vi "About.vi"() -> ()   [LabVIEW 2015]
uses:
  <vilib>/Platform/browser.llb/Open URL in Default Browser (string).vi
  GlobalVar.vi
panel:
  in  "btnReg":bool
  out "txtCopyright":string="版权归许晓通所有,欢迎个人转发分享。"
  out "txtContact":string="如有其它疑问，欢迎私信留言或联系QQ：19627152   QQ群：646900507。"
  out "txtXCANdeveloper":string="作者：Jay Sur (许晓通) @华南理工大学"
  out "txtXCAN":string="X-CAN离线分析平台"
  out "JayWeb":string
  in  "GoJayWeb":bool
  out "txtshowSupportFormat":string caption="The file format supported:"
  in  "btnGoBlog":bool
  in  "btnClose":bool
  out "UserGroup":string caption="用户组:"
  out "CurVersion":string caption="Version:"
  out "HelpBlogURL":string caption="Introduction and help, please see:"
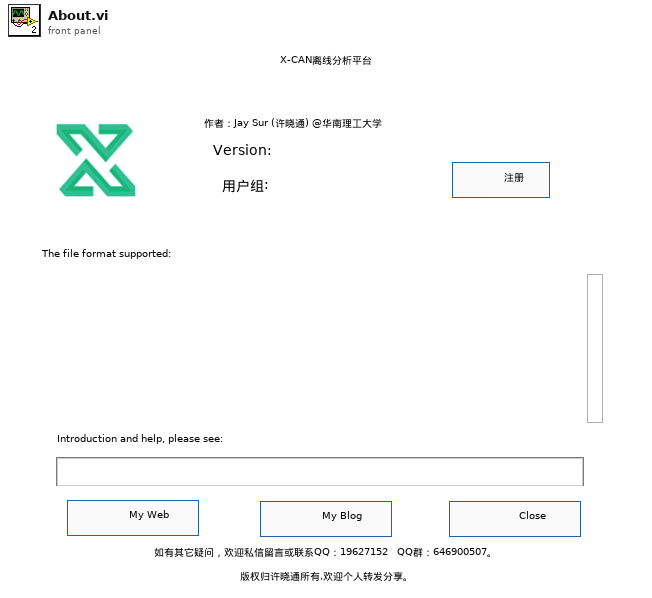
[diagram p1: front panel]
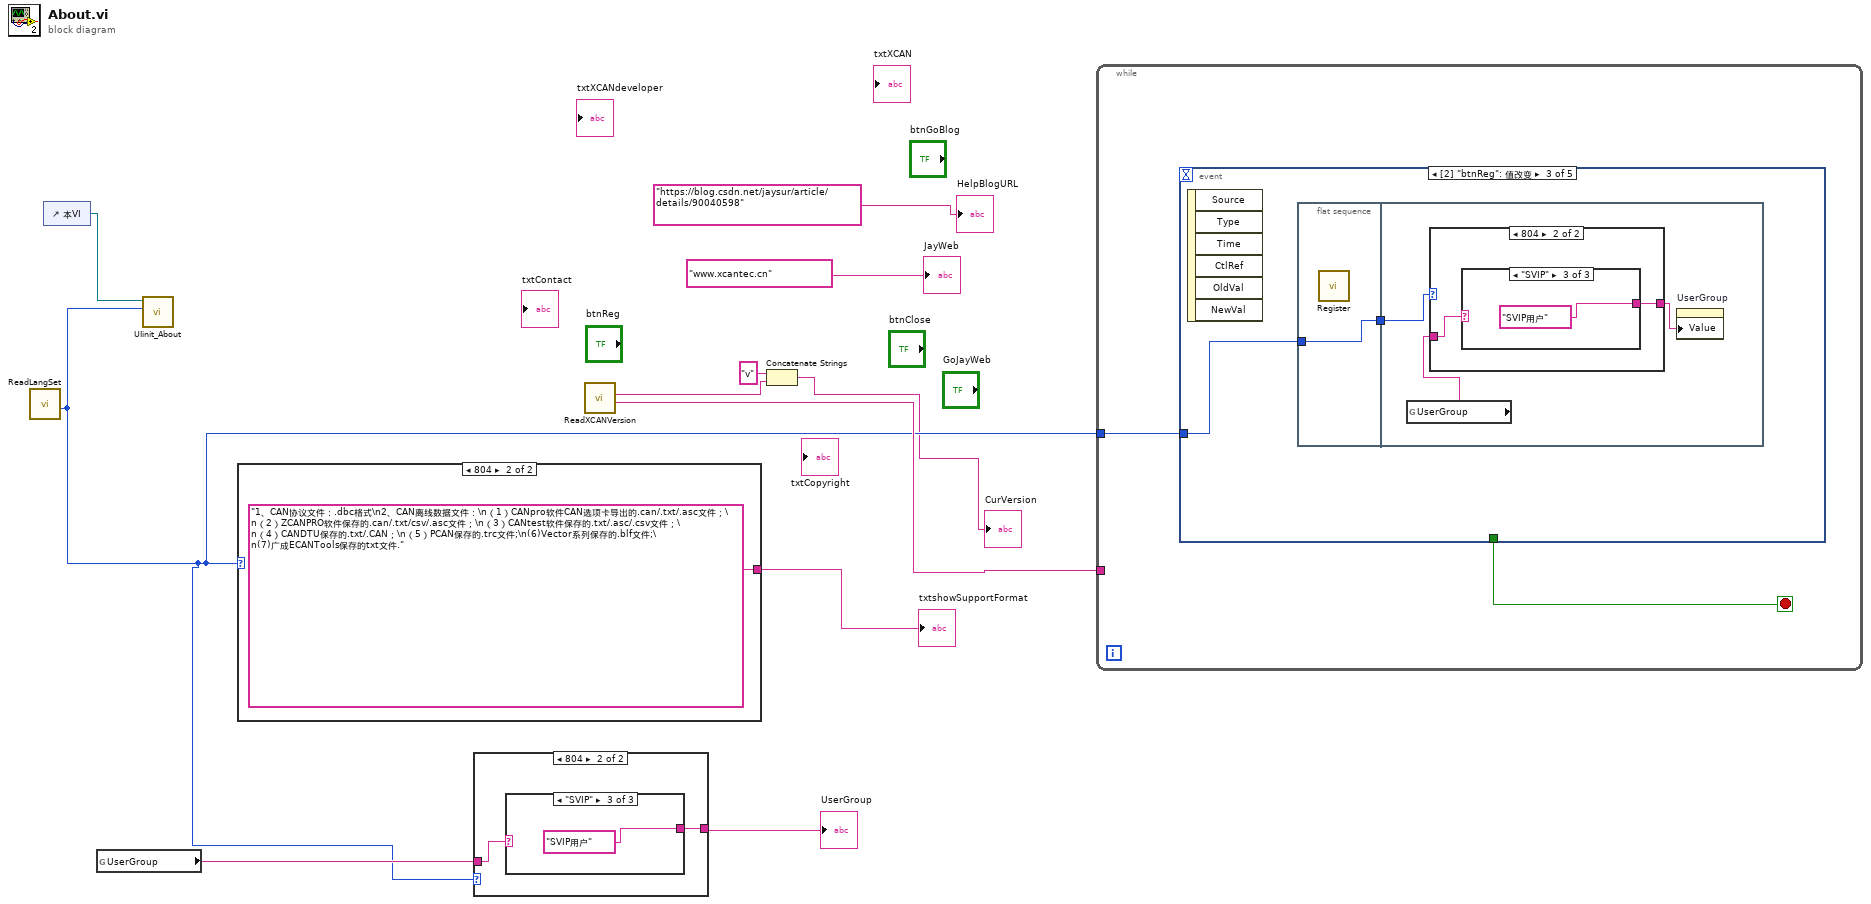
[diagram p0: block diagram]
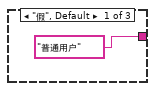
[diagram p3: hidden frame]
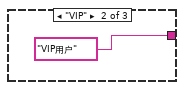
[diagram p4: hidden frame]
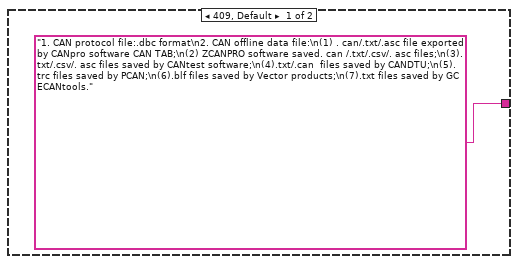
[diagram p5: hidden frame]
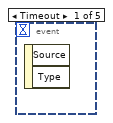
[diagram p6: hidden frame]
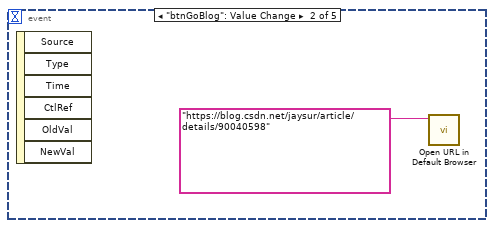
[diagram p7: hidden frame]
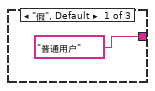
[diagram p9: hidden frame]
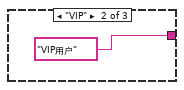
[diagram p10: hidden frame]
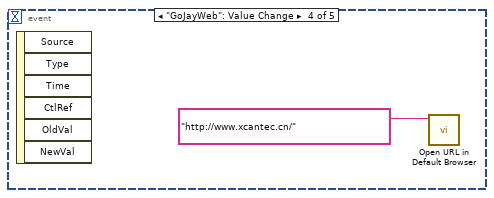
[diagram p11: hidden frame]
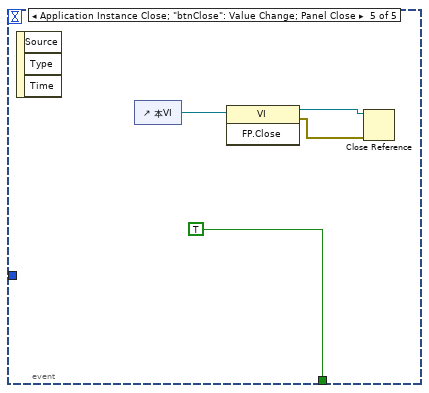
[diagram p12: hidden frame]
diagram:
  n1 = call "ReadLangSet.vi"() -> ("Language"=w6:u32)  [unwired: 11 in]
  n2 = control-ref of="本VI"() -> (w10:refnum<vi>)
  n3 = global read "GlobalVar.vi" "UserGroup"() -> (w7:string)
  n4 = call "UIinit_About.vi"("Language"=w6, "VI输入"=w10) -> ()  [unwired: 10 in]
  n5 = case shown="804" w6 {
    tunnel: ["1. CAN protocol file:.dbc format\n2. CAN offline data file:\n(1) . can/.txt/.asc file exported by CANpro software CAN TAB;\n(2) ZCANPRO software saved. can /.txt/.csv/. asc files;\n(3).txt/.csv/. asc files saved by CANtest software;\n(4).txt/.can  files saved by CANDTU;\n(5).trc files saved by PCAN;\n(6).blf files saved by Vector products;\n(7).txt files saved by GC ECANtools." "1、CAN协议文件：.dbc格式\n2、CAN离线数据文件：\n（1）CANpro软件CAN选项卡导出的.can/.txt/.asc文件；\n（2）ZCANPRO软件保存的.can/.txt/csv/.asc文件；\n（3）CANtest软件保存的.txt/.asc/.csv文件；\n（4）CANDTU保存的.txt/.CAN；\n（5）PCAN保存的.trc文件;\n(6)Vector系列保存的.blf文件;\n(7)广成ECANTools保存的txt文件." ("软件介绍及使用帮助，请看：")] -> w5
    frame 409, Default {
    }
    frame 804 {
    }
  }
  "txtshowSupportFormat" <- w5
  n6 = case shown="804" w6 {
    tunnel: [w14 w15] -> w2
    tunnel: w7 -> [w14 w16]
    frame 409, Default {
    }
    frame 804 {
      n7 = case shown="\"SVIP\"" w16 {
        tunnel: ["普通用户" "VIP用户" "SVIP用户"] -> w15
        frame "假", Default {
        }
        frame "VIP" {
        }
        frame "SVIP" {
        }
      }
    }
  }
  "UserGroup" <- w2
  n8 = call "ReadXCANVersion.vi"() -> ("InstallTime"=w11:string, "Version"=w8:string)  [unwired: 9 in]
  n9 = Concatenate Strings("v" ("字符串"), w8) -> (→"CurVersion":string)
  n10 = while {
    tunnel: w11 -> [_]
    tunnel: w6 -> [w20]
    stop <- w21 stop-if-true
    n11 = event shown="[2] \"btnReg\": 值改变" {
      selector: _ -> [_ _ _ _ _]
      dyn-events: _ -> [_ _ _ _ _]
      timeout: _ -> [_ _ _ _ _]
      tunnel: [_ _ _ _ TRUE] -> w21
      tunnel: w20 -> [_ _ w24 _ _]
      event Timeout {
        n12 = event-data() -> ()  [unwired: 1 in, 2 out]
      }
      event "btnGoBlog": Value Change {
        n13 = event-data() -> ()  [unwired: 1 in, 6 out]
        n14 = call-poly <vilib>:"Open URL in Default Browser.vi"("URL"="https://blog.csdn.net/jaysur/article/details/90040598") -> ()  [unwired: 5 in, 2 out]
      }
      event "btnReg": Value Change {
        n15 = event-data() -> ()  [unwired: 1 in, 6 out]
        n16 = flat-sequence {
          tunnel: w24 -> [w25]
          tunnel: [w25] -> w23
          tunnel: w23 -> [w27]
          frame #0 {
            n17 = call "Register.vi"() -> ()  [unwired: 12 in]
          }
          frame #1 {
            n18 = global read "GlobalVar.vi" "UserGroup"() -> (w26:string)
            n19 = case shown="804" w27 {
              tunnel: [w29 w30] -> w28
              tunnel: w26 -> [w29 w31]
              frame 409, Default {
              }
              frame 804 {
                n20 = case shown="\"SVIP\"" w31 {
                  tunnel: ["普通用户" "VIP用户" "SVIP用户"] -> w30
                  frame "假", Default {
                  }
                  frame "VIP" {
                  }
                  frame "SVIP" {
                  }
                }
              }
            }
            n21 = property on="UserGroup" class="Str"("Value"=w28) -> ()  [unwired: 2 in, 2 out]
          }
        }
      }
      event "GoJayWeb": Value Change {
        n22 = event-data() -> ()  [unwired: 1 in, 6 out]
        n23 = call-poly <vilib>:"Open URL in Default Browser.vi"("URL"="http://www.xcantec.cn/") -> ()  [unwired: 5 in, 2 out]
      }
      event Application Instance Close; "btnClose": Value Change; Panel Close {
        n24 = event-data() -> ()  [unwired: 1 in, 3 out]
        n25 = control-ref of="本VI"() -> (w38:refnum<vi>)
        n26 = invoke class="VI" method="FP.Close"(reference=w38) -> (reference out=w37:refnum<vi>, error out=w36:errorcluster)  [unwired: 2 in, 1 out]
        n27 = Close Reference(reference=w37, error in (no error)=w36) -> ()  [unwired: 1 out]
      }
    }
  }
  "HelpBlogURL" <- "https://blog.csdn.net/jaysur/article/details/90040598" ("软件介绍及使用帮助，请看：")
  "JayWeb" <- "www.xcantec.cn" ("URL")
